vi "OXYGEN_FGV_MeasurementValues.vi"(7 "Mode":T2, 8 "error in (no error)":errorcluster, 11 "Common Refs":T1={"LBox_ChList"=refnum, "STR_LoggingChName1"=refnum, "Listbox_ChValue"=refnum, "STR_LoggingChName2"=refnum, "STR_LoggingChName3"=refnum, "STR_LoggingChName4"=refnum, "STR_LoggingChName5"=refnum, "STR_LoggingChName6"=refnum, "OXY_SCPI Ref"="TCPIP0::192.168.1.75::10001::SOCKET", "STR_ChName1"=refnum, "STR_ChName2"=refnum, "STR_ChName3"=refnum, "STR_ChName4"=refnum, "STR_ChName5"=refnum, "STR_ChName6"=refnum, "Enum_SelectTimestampFormat"=refnum, "GRAPH-XY_ELOG"=refnum, "GRAPH-XY_Measurement"=refnum, "Button_StartBuffer"=refnum, "Button_StopBuffer"=refnum, "Button_FetchData"=refnum, "STR_LoggingChName1"=refnum, "STR_LoggingChName2"=refnum, "STR_LoggingChName3"=refnum, "STR_LoggingChName4"=refnum, "STR_LoggingChName5"=refnum, "STR_LoggingChName6"=refnum, "Enum_SelectCalc"=refnum, "Num_SetDurationTime"=refnum, "Button_StopTransfer"=refnum, "Button_StartTransfer"=refnum, "STR_IN_AggregationRate"=refnum, "Button_Disconnect"=refnum, "Button_Connect"=refnum, "Button_StartRec"=refnum, "Button_PauseRec"=refnum, "Button_StopRec"=refnum, "Bool_StatusLED"=refnum, "Indicator_RecordingStatus"=refnum}) -> (0 "error in (no error)":errorcluster, 1 "Value List":dbl[](array[numeric]))   [LabVIEW 2018]
uses:
  TypeDefs/TD_Case_MeasurementValues.ctl
  TypeDefs/Refs_Common.ctl
  TypeDefs/Graph_DataArrayElement.ctl
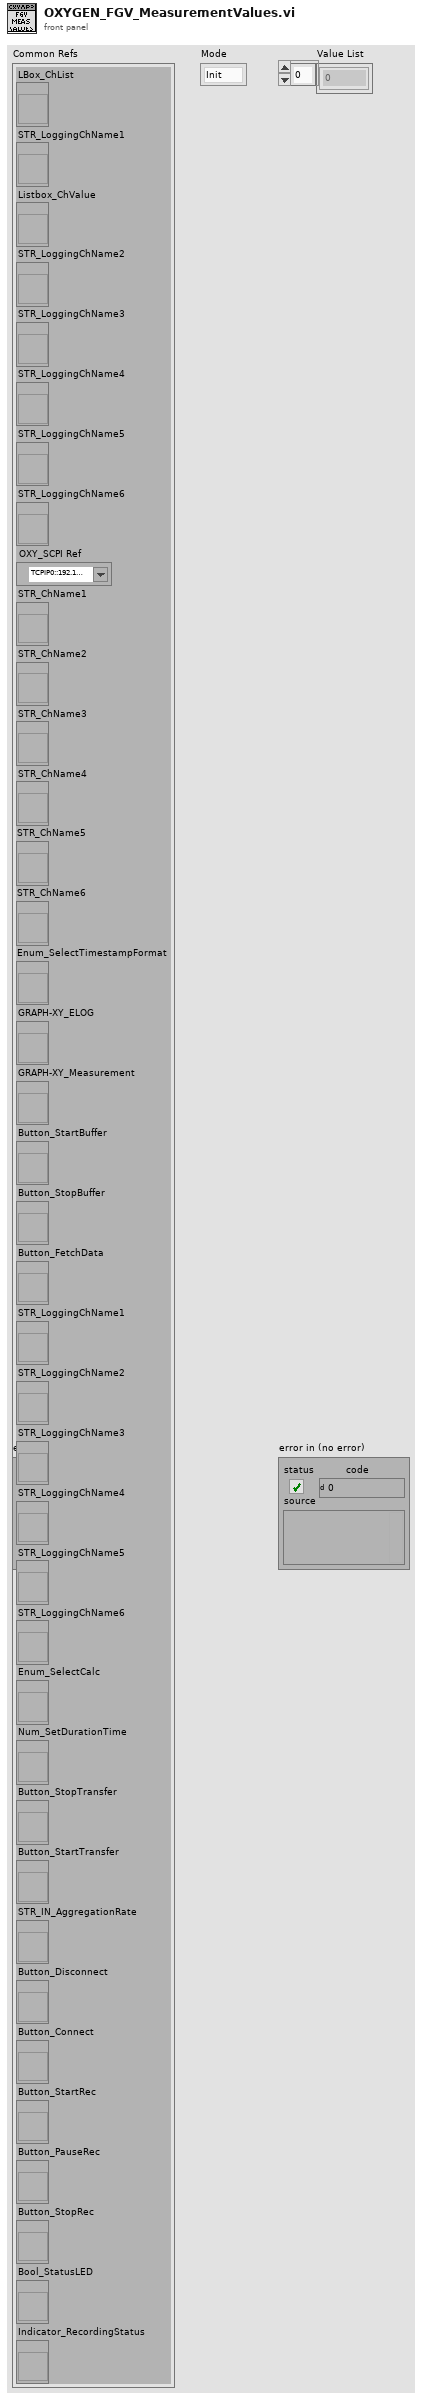
[diagram p1: front panel]
types:
  T1 = typedef "Refs_Common.ctl" = cluster{"LBox_ChList":refnum<vi>, "STR_LoggingChName1":refnum<vi>, "Listbox_ChValue":refnum<vi>, "STR_LoggingChName2":refnum<vi>, "STR_LoggingChName3":refnum<vi>, "STR_LoggingChName4":refnum<vi>, "STR_LoggingChName5":refnum<vi>, "STR_LoggingChName6":refnum<vi>, "OXY_SCPI Ref":refnum<visa-resource-name>, "STR_ChName1":refnum<vi>, "STR_ChName2":refnum<vi>, "STR_ChName3":refnum<vi>, "STR_ChName4":refnum<vi>, "STR_ChName5":refnum<vi>, "STR_ChName6":refnum<vi>, "Enum_SelectTimestampFormat":refnum<vi>, "GRAPH-XY_ELOG":refnum<vi>, "GRAPH-XY_Measurement":refnum<vi>, "Button_StartBuffer":refnum<vi>, "Button_StopBuffer":refnum<vi>, "Button_FetchData":refnum<vi>, "STR_LoggingChName1":refnum<vi>, "STR_LoggingChName2":refnum<vi>, "STR_LoggingChName3":refnum<vi>, "STR_LoggingChName4":refnum<vi>, "STR_LoggingChName5":refnum<vi>, "STR_LoggingChName6":refnum<vi>, "Enum_SelectCalc":refnum<vi>, "Num_SetDurationTime":refnum<vi>, "Button_StopTransfer":refnum<vi>, "Button_StartTransfer":refnum<vi>, "STR_IN_AggregationRate":refnum<vi>, "Button_Disconnect":refnum<vi>, "Button_Connect":refnum<vi>, "Button_StartRec":refnum<vi>, "Button_PauseRec":refnum<vi>, "Button_StopRec":refnum<vi>, "Bool_StatusLED":refnum<vi>, "Indicator_RecordingStatus":refnum<vi>}
  T2 = typedef "TD_Case_MeasurementValues.ctl" = enum16{"Init", "Start", "Stop", "ChangeChannel", "Refresh"}
  T3 = enum8{"Enabled", "Disabled", "Disabled and Grayed Out"}
  T4 = typedef "Graph_DataArrayElement.ctl" = cluster{"Timestamp":timestamp[], "Value":dbl[]}
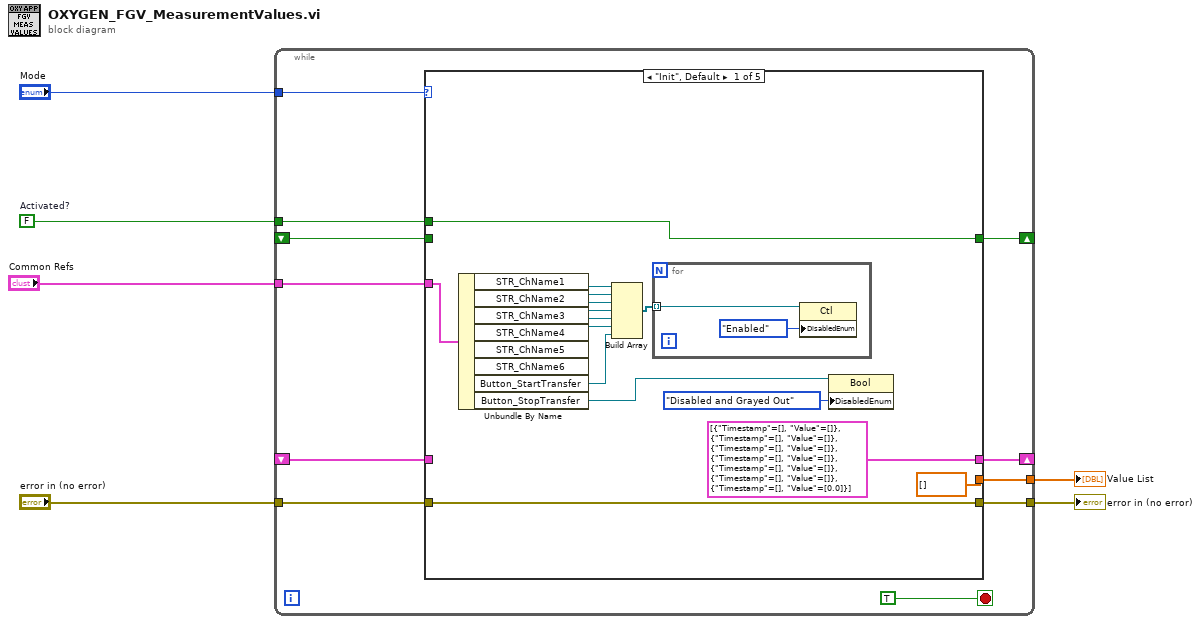
[diagram p0: block diagram]
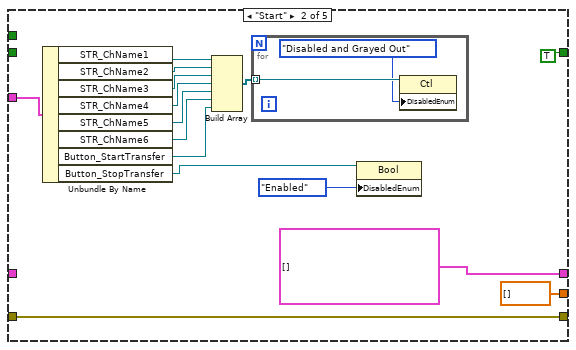
[diagram p2: hidden frame]
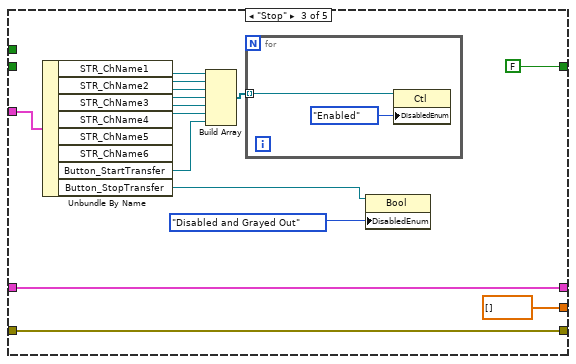
[diagram p3: hidden frame]
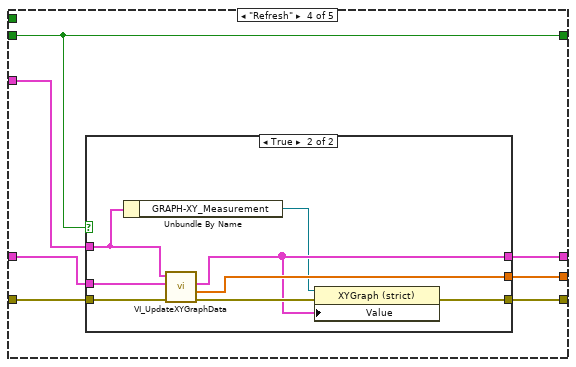
[diagram p4: hidden frame]
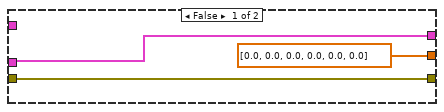
[diagram p5: hidden frame]
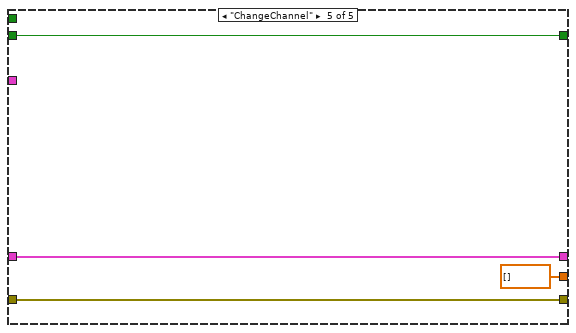
[diagram p6: hidden frame]
diagram:
  w5 = FALSE  # Activated?
  n1 = while {
    tunnel: "Mode" -> [w16]
    tunnel: w5 -> [w15]
    shift-right: [w14] -> _
    shift-left: _ -> [w13]
    tunnel: [w12] -> w4
    tunnel: "error in (no error)" -> [w11]
    shift-right: [w9] -> _
    shift-left: _ -> [w10]
    tunnel: [w8] -> w2
    tunnel: "Common Refs" -> [w7]
    stop <- TRUE stop-if-true
    n2 = case shown="\"Init\", Default" w16 {
      tunnel: w15 -> [w32 _ _ _ _]
      tunnel: [w32 TRUE ("Activated?") FALSE ("Activated?") w71 w90] -> w14
      tunnel: w13 -> [_ _ _ w71 w90]
      tunnel: [w31 w48 w64 w74 w89] -> w12
      tunnel: w11 -> [w31 w48 w64 w75 w89]
      tunnel: w10 -> [_ _ w65 w73 w88]
      tunnel: [T4[] [{"Timestamp"=[], "Value"=[]}, {"Timestamp"=[], "Value"=[]}, {"Timestamp"=[], "Value"=[]}, {"Timestamp"=[], "Value"=[]}, {"Timestamp"=[], "Value"=[]}, {"Timestamp"=[], "Value"=[]}, {"Timestamp"=[], "Value"=[0.0]}] ("Updated Graph Data") T4[] [] ("Updated Graph Data") w65 w72 w88] -> w9
      tunnel: [dbl[] [] ("Value List") dbl[] [] ("Value List") dbl[] [] ("Value List") w70 dbl[] [] ("Value List")] -> w8
      tunnel: w7 -> [w22 w46 w55 w69 _]
      frame "Init", Default {
        n3 = Unbundle By Name(w22) -> ("STR_ChName1"=w29:refnum<vi>, "STR_ChName2"=w28:refnum<vi>, "STR_ChName3"=w27:refnum<vi>, "STR_ChName4"=w26:refnum<vi>, "STR_ChName5"=w25:refnum<vi>, "STR_ChName6"=w24:refnum<vi>, "Button_StartTransfer"=w20:refnum<vi>, "Button_StopTransfer"=w18:refnum<vi>)
        n4 = Build Array(w29, w28, w27, w26, w25, w24, w20) -> (w23:refnum<vi>[])
        n5 = for {
          tunnel: w23 -> [w34] mode=indexing
          n6 = property class="Ctl"(reference=w34, "DisabledEnum"=T3."Enabled" ("Disabled")) -> ()  [unwired: 1 in, 2 out]
        }
        n7 = property class="Bool"(reference=w18, "DisabledEnum"=T3."Disabled and Grayed Out" ("Disabled")) -> ()  [unwired: 1 in, 2 out]
      }
      frame "Start" {
        n8 = Unbundle By Name(w46) -> ("STR_ChName1"=w45:refnum<vi>, "STR_ChName2"=w44:refnum<vi>, "STR_ChName3"=w43:refnum<vi>, "STR_ChName4"=w42:refnum<vi>, "STR_ChName5"=w41:refnum<vi>, "STR_ChName6"=w40:refnum<vi>, "Button_StartTransfer"=w35:refnum<vi>, "Button_StopTransfer"=w36:refnum<vi>)
        n9 = Build Array(w45, w44, w43, w42, w41, w40, w35) -> (w39:refnum<vi>[])
        n10 = for {
          tunnel: w39 -> [w51] mode=indexing
          n11 = property class="Ctl"(reference=w51, "DisabledEnum"=T3."Disabled and Grayed Out" ("Disabled")) -> ()  [unwired: 1 in, 2 out]
        }
        n12 = property class="Bool"(reference=w36, "DisabledEnum"=T3."Enabled" ("Disabled")) -> ()  [unwired: 1 in, 2 out]
      }
      frame "Stop" {
        n13 = Unbundle By Name(w55) -> ("STR_ChName1"=w56:refnum<vi>, "STR_ChName2"=w57:refnum<vi>, "STR_ChName3"=w58:refnum<vi>, "STR_ChName4"=w59:refnum<vi>, "STR_ChName5"=w60:refnum<vi>, "STR_ChName6"=w61:refnum<vi>, "Button_StartTransfer"=w54:refnum<vi>, "Button_StopTransfer"=w52:refnum<vi>)
        n14 = Build Array(w56, w57, w58, w59, w60, w61, w54) -> (w62:refnum<vi>[])
        n15 = for {
          tunnel: w62 -> [w68] mode=indexing
          n16 = property class="Ctl"(reference=w68, "DisabledEnum"=T3."Enabled" ("Disabled")) -> ()  [unwired: 1 in, 2 out]
        }
        n17 = property class="Bool"(reference=w52, "DisabledEnum"=T3."Disabled and Grayed Out" ("Disabled")) -> ()  [unwired: 1 in, 2 out]
      }
      frame "Refresh" {
        n18 = case shown="True" w71 {
          tunnel: w75 -> [w77 w86]
          tunnel: [w77 w84] -> w74
          tunnel: w73 -> [w78 w83]
          tunnel: [w78 w81] -> w72
          tunnel: [dbl[] [0.0, 0.0, 0.0, 0.0, 0.0, 0.0] ("Value List") w82] -> w70
          tunnel: w69 -> [_ w80]
          frame False {
          }
          frame True {
            n19 = Unbundle By Name(w80) -> ("GRAPH-XY_Measurement"=w79:refnum<vi>)
            n20 = call "VI_UpdateXYGraphData.vi"("error in (no error)"=w86, "Old Graph Data"=w83, "Common Refs"=w80) -> ("error out"=w85:errorcluster, "Latest Value per Item"=w82:dbl[], "Updated Graph Data"=w81:T4[])  [unwired: 6 in]
            n21 = property class="XYGraph (strict)"(reference=w79, error in=w85, "Value"=w81) -> (error out=w84:errorcluster)  [unwired: 1 out]
          }
        }
      }
      frame "ChangeChannel" {
      }
    }
  }
  "error in (no error)" <- w4
  "Value List" <- w2
